vi "Run.vi"(8 "error in (no error)":errorcluster, 9 "Penalty":dbl, 10 "Maze":i32[][](array[numeric]), 11 "Runner in":refnum<class "Cross.lvclass">) -> (0 "error out":errorcluster, 1 "Direction":T1, 2 "Action":T2, 3 "Runner out":refnum<class "Cross.lvclass">, 4 "Replicated":refnum<class "Square.lvclass">)   [LabVIEW 2015, in "Cross.lvclass"]
uses:
  Cross.lvclass
  Type Defs/Action Enum.ctl
  Type Defs/Direction Enum.ctl
  Square/Square.lvclass
  Cross.lvclass/Cross.ctl
  Type Defs/SB Type Defs.lvlib
  Carl/Common/Common.lvlib
panel:
  # "NOTICE - YOU MUST NOT REMOVE THIS NOTICE. PER THE FOLLOWING LICENSE, YOU MAY REPRODUCE THIS SOFTWARE PROVIDED YOU FOLLOW THE TERMS\nOF THE LICENSE.\n\n---BEGIN BSD LICENSE (http://opensource.org/licenses/BSD-2-Clause)---\nCopyright (c) 2015, Endigit, Inc. <robert@endigit.com>\nAll rights reserved.\n\nRedistribution and use in source and binary forms, with or without modification, are permitted provided that the following conditions are met:\n\n1. Redistributions of source code must retain the above copyright notice, this list of conditions and the following disclaimer.\n\n2. Redistributions in binary form must reproduce the above copyright notice, this list of conditions and the following disclaimer in the documentation and/or other \nmaterials provided with the distribution.\n\nTHIS SOFTWARE IS PROVIDED BY THE COPYRIGHT HOLDERS AND CONTRIBUTORS \"AS IS\" AND ANY EXPRESS OR IMPLIED WARRANTIES, INCLUDING, BUT NOT \nLIMITED TO, THE IMPLIED WARRANTIES OF MERCHANTABILITY AND FITNESS FOR A PARTICULAR PURPOSE ARE DISCLAIMED. IN NO EVENT SHALL THE COPYRIGHT \nHOLDER OR CONTRIBUTORS BE LIABLE FOR ANY DIRECT, INDIRECT, INCIDENTAL, SPECIAL, EXEMPLARY, OR CONSEQUENTIAL DAMAGES (INCLUDING, BUT NOT \nLIMITED TO, PROCUREMENT OF SUBSTITUTE GOODS OR SERVICES; LOSS OF USE, DATA, OR PROFITS; OR BUSINESS INTERRUPTION) HOWEVER CAUSED AND ON \nANY THEORY OF LIABILITY, WHETHER IN CONTRACT, STRICT LIABILITY, OR TORT (INCLUDING NEGLIGENCE OR OTHERWISE) ARISING IN ANY WAY OUT OF THE USE \nOF THIS SOFTWARE, EVEN IF ADVISED OF THE POSSIBILITY OF SUCH DAMAGE.\n---END BSD LICENSE---"
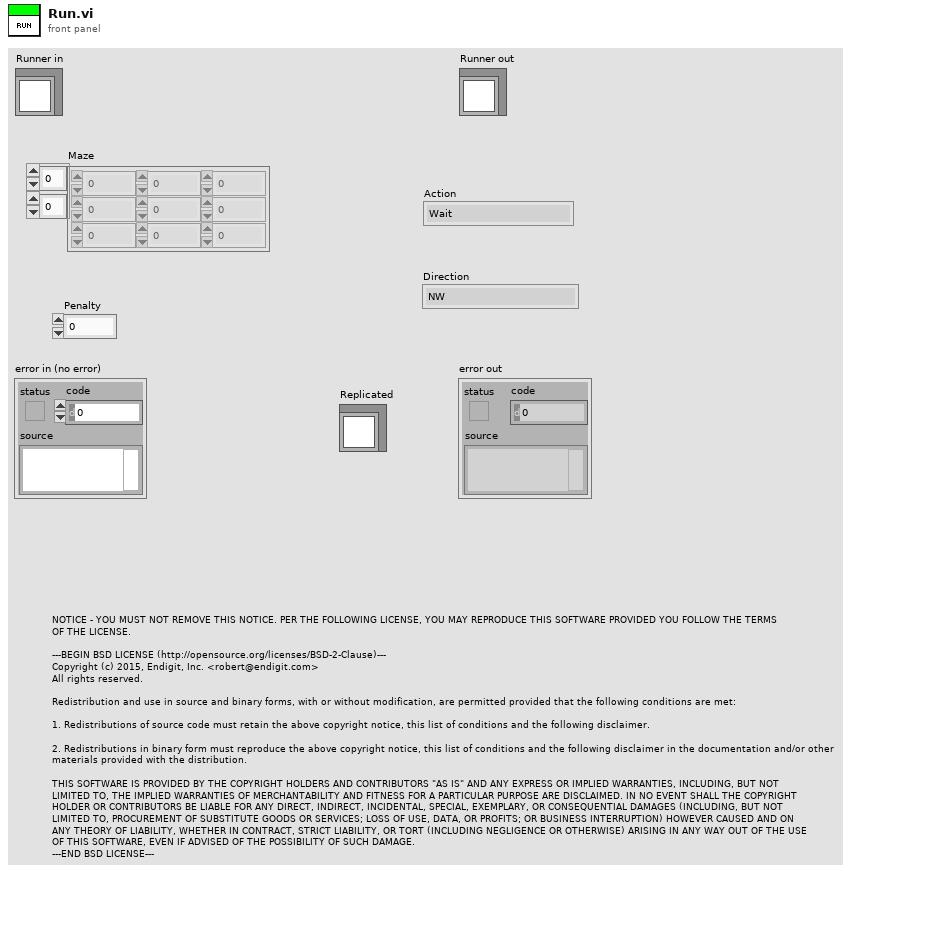
[diagram p1: front panel]
types:
  T1 = typedef "SB Type Defs.lvlib/Direction Enum.ctl" = enum16{"NW", "N", "NE", "E", "SE", "S", "SW", "W"}
  T2 = typedef "SB Type Defs.lvlib/Action Enum.ctl" = enum16{"Wait", "Move", "Attack", "Replicate"}
  T3 = enum16{"Raw", "Spawner", "Builder", "Gunner", "Fighter"}
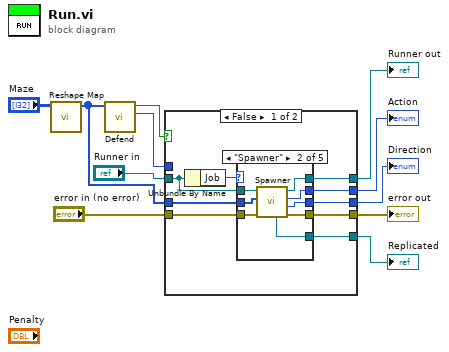
[diagram p0: block diagram]
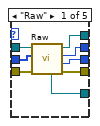
[diagram p2: hidden frame]
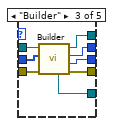
[diagram p3: hidden frame]
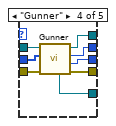
[diagram p4: hidden frame]
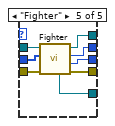
[diagram p5: hidden frame]
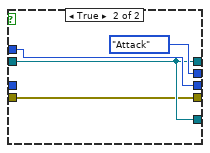
[diagram p6: hidden frame]
diagram:
  n1 = call "Reshape Map.vi"("Maze (0: Empty, -1: Enemy. >0: Teammate"="Maze") -> ("Map"=w1:i32[])  [unwired: 9 in, 1 out]
  n2 = call "Defend.vi"("Maze"=w1) -> ("Direction"=w11:T1, "Defend?"=w10:bool)  [unwired: 9 in]
  n3 = case shown="False" w10 {
    tunnel: w1 -> [w14 _]
    tunnel: w11 -> [_ w63]
    tunnel: "Runner in" -> [w20 w62]
    tunnel: [w18 Action_Enum."Attack" ("Action")] -> w8
    tunnel: [w17 w63] -> w7
    tunnel: [w16 w62] -> w6
    tunnel: [w15 w62] -> w3
    tunnel: "error in (no error)" -> [w13 w61]
    tunnel: [w12 w61] -> w4
    frame False {
      n4 = Unbundle By Name(w20) -> ("Job"=w19:T3)
      n5 = case shown="\"Spawner\"" w19 {
        tunnel: w20 -> [w28 w36 w37 w45 w53]
        tunnel: [w22 w30 w43 w51 w59] -> w18
        tunnel: [w21 w31 w42 w50 w58] -> w17
        tunnel: [w24 w29 w44 w52 w60] -> w16
        tunnel: [w25 w34 w40 w48 w56] -> w15
        tunnel: w14 -> [w27 w35 w38 w46 w54]
        tunnel: w13 -> [w26 w33 w39 w47 w55]
        tunnel: [w23 w32 w41 w49 w57] -> w12
        frame "Raw" {
          n6 = call "Raw.vi"("error in (no error)"=w26, "Map"=w27, "Raw In"=w28) -> ("error out"=w23:errorcluster, "Direction"=w21:T1, "Action"=w22:T2, "Raw Out"=w24:refnum<class "Cross.lvclass">, "Replicated Class"=w25:refnum<class "Cross.lvclass">)  [unwired: 4 in]
        }
        frame "Spawner" {
          n7 = call "Spawner.vi"("error in (no error)"=w33, "Map"=w35, "Spawner In"=w36) -> ("error out"=w32:errorcluster, "Direction"=w31:T1, "Action"=w30:T2, "Spawner Out"=w29:refnum<class "Cross.lvclass">, "Replicated Class"=w34:refnum<class "Cross.lvclass">)  [unwired: 4 in]
        }
        frame "Builder" {
          n8 = call "Builder.vi"("error in (no error)"=w39, "Map"=w38, "Builder In"=w37) -> ("error out"=w41:errorcluster, "Direction"=w42:T1, "Action"=w43:T2, "Builder Out"=w44:refnum<class "Cross.lvclass">, "Replicated Class"=w40:refnum<class "Cross.lvclass">)  [unwired: 4 in]
        }
        frame "Gunner" {
          n9 = call "Gunner.vi"("error in (no error)"=w47, "Map"=w46, "Gunner In"=w45) -> ("error out"=w49:errorcluster, "Direction"=w50:T1, "Action"=w51:T2, "Gunner Out"=w52:refnum<class "Cross.lvclass">, "Replicated Class"=w48:refnum<class "Cross.lvclass">)  [unwired: 4 in]
        }
        frame "Fighter" {
          n10 = call "Fighter.vi"("error in (no error)"=w55, "Map"=w54, "Fighter In"=w53) -> ("error out"=w57:errorcluster, "Direction"=w58:T1, "Action"=w59:T2, "Fighter Out"=w60:refnum<class "Cross.lvclass">, "Replicated Class"=w56:refnum<class "Cross.lvclass">)  [unwired: 4 in]
        }
      }
    }
    frame True {
    }
  }
  "error out" <- w4
  "Runner out" <- w6
  "Action" <- w8
  "Direction" <- w7
  "Replicated" <- w3
